vi "总磷单步调试对话框.vi"() -> ()   [LabVIEW 2016, in "斯坦道总磷总氮.lvlib"]
panel:
  in  "单步调试":T9={"注射泵"=enum."注入", "阀口选择"=enum."V1", "灯"=enum."未选择", "ADC值"=enum."未选择", "数值"=4000, "项目输入"=0, "控温"={"氨氮控温"=FALSE, "消解"=FALSE, "恒温"=FALSE, "降温"=FALSE}, "外设选择"={"蠕动泵"=FALSE, "电磁阀1"=FALSE, "电磁阀2"=FALSE, "慢速"=FALSE}, "外设选择2"={"V9-1"=FALSE, "V9-2"=FALSE, "顺时针"=FALSE, "逆时针"=FALSE}, "反滴定"=FALSE, "试剂检测"=FALSE}
  in  "停止":bool
  out "注射器温度":sgl
  out "消解温度":sgl
  out "ADC":sgl
  out "F3":sgl format="%#.6f"
  out "F2":sgl format="%#.6f"
  out "F1":sgl format="%#.6f"
  out "F0":sgl format="%#.6f"
  in  "退出":bool
  in  "启动":bool
  # "单步调试界面"
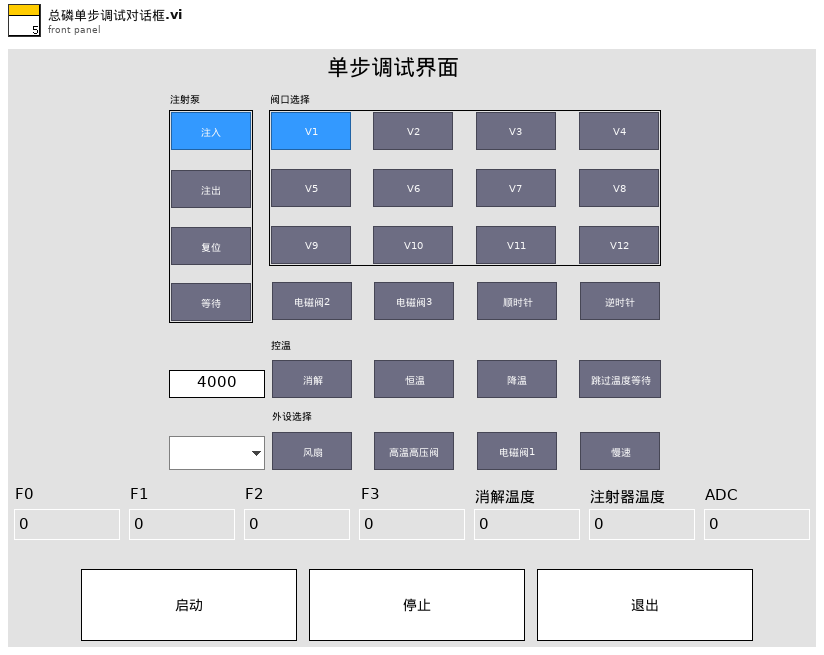
[diagram p1: front panel]
types:
  T1 = typedef "SingleStepTestV3.lvlib/SingleStepTestV3.lvclass/注射泵操作.ctl" = enum32{"复位", "注入", "注出", "等待"}
  T2 = typedef "SingleStepTestV3.lvlib/SingleStepTestV3.lvclass/阀口操作.ctl" = enum32{"未选择", "V1", "V2", "V3", "V4", "V5", "V6", "V7", "V8", "V9", "V10", "V11", "V12"}
  T3 = typedef "SingleStepTestV3.lvlib/SingleStepTestV3.lvclass/灯选择.ctl" = enum32{"未选择", "365", "520", "660", "氙灯/紫灯"}
  T4 = typedef "SingleStepTestV3.lvlib/SingleStepTestV3.lvclass/ADC选择.ctl" = enum32{"未选择", "ADC365", "ADC520", "ADC660", "光谱仪"}
  T5 = typedef "SingleStepTestV3.lvlib/SingleStepTestV3.lvclass/控温操作.ctl" = cluster{"氨氮控温":bool, "消解":bool, "恒温":bool, "降温":bool}
  T6 = typedef "SingleStepTestV3.lvlib/SingleStepTestV3.lvclass/外设选择.ctl" = cluster{"蠕动泵":bool, "电磁阀1":bool, "电磁阀2":bool, "慢速":bool}
  T7 = typedef "SingleStepTestV3.lvlib/SingleStepTestV3.lvclass/外设选择2.ctl" = cluster{"V9-1":bool, "V9-2":bool, "顺时针":bool, "逆时针":bool}
  T8 = typedef "SingleStepTestV3.lvlib/SingleStepTestV3.lvclass/布尔按钮.ctl" = bool
  T9 = cluster{"注射泵":T1, "阀口选择":T2, "灯":T3, "ADC值":T4, "数值":i16, "项目输入":u16, "控温":T5, "外设选择":T6, "外设选择2":T7, "反滴定":T8, "试剂检测":T8}
  T10 = typedef "SingleStepTestV3.lvlib/SingleStepTestV3.lvclass/仪器版本.ctl" = enum16{"V3.1版", "V4版", "V3版", "V4.2版"}
  T11 = typedef "操作日志字段定义.ctl" = cluster{"时间":timestamp, "参数":string, "日志信息":string, "流程参数":string}
  T12 = cluster{"系统时间":timestamp, "工作状态":u16, "测量模式":enum16{"待机", "连续模式", "周期模式", "定点模式", "受控模式", "手动模式"}, "告警代码":u16, "故障代码":u16, "日志代码":u16, "软件版本":u16, "F0":sgl, "F1":sgl, "F2":sgl, "F3":sgl, "T":sgl, "H":sgl, "id":u16, "flowid":u16, "量程":u16, "总磷控温温度1":sgl, "营养盐控温温度2":sgl, "ADC":sgl, "结果值":sgl, "运行时间":u16, "步骤详情":string, "步骤流程":string}
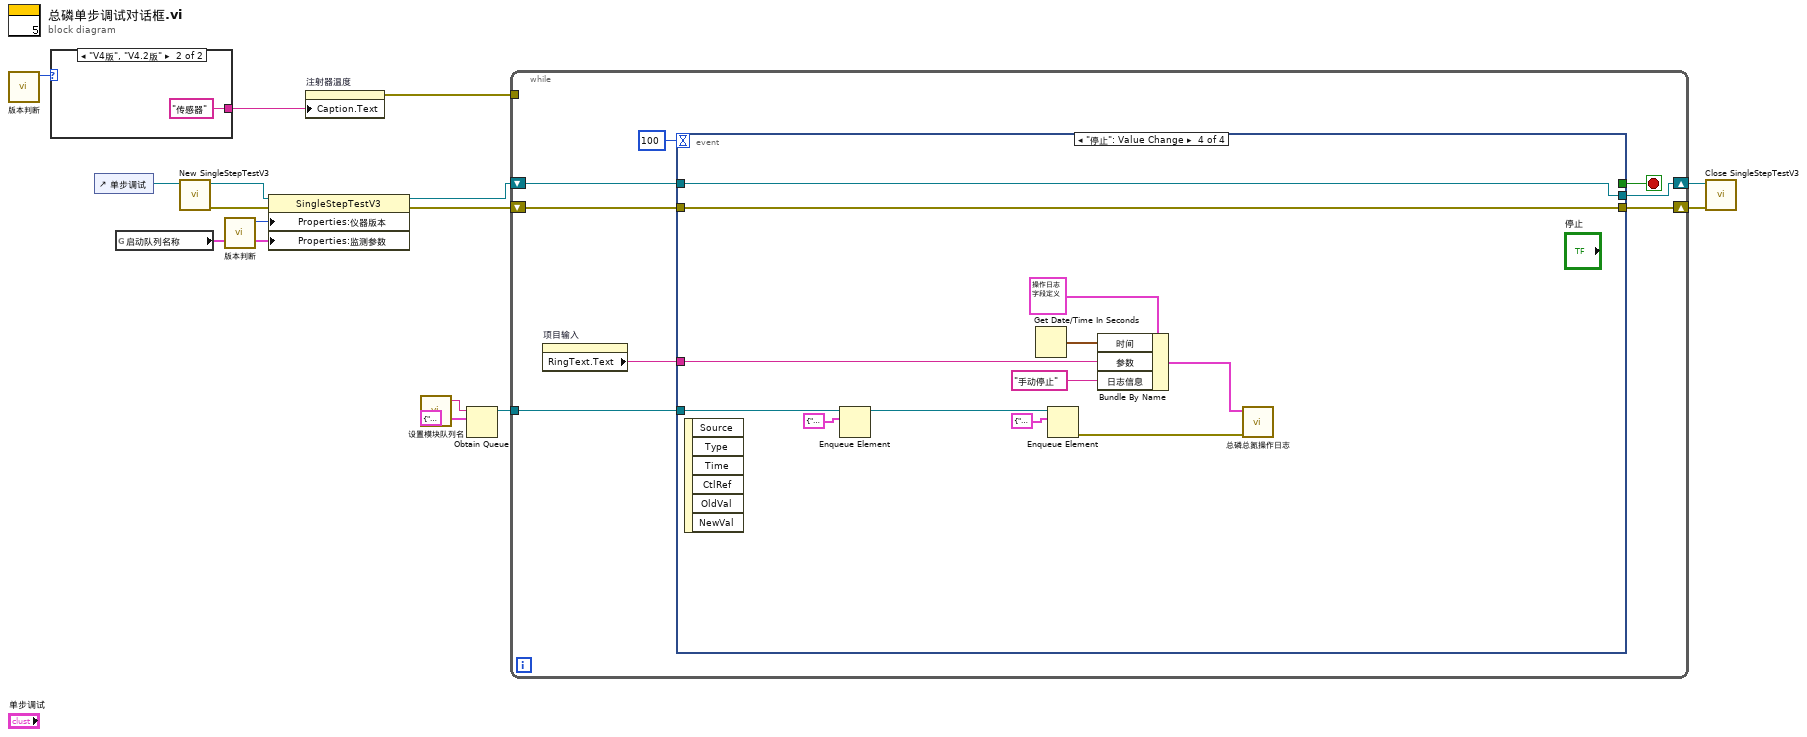
[diagram p0: block diagram]
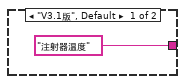
[diagram p2: hidden frame]
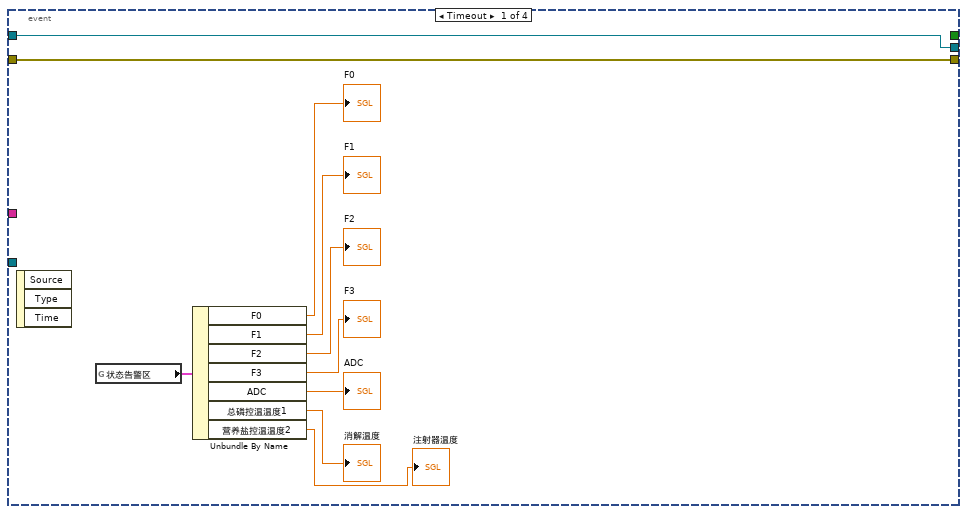
[diagram p3: hidden frame]
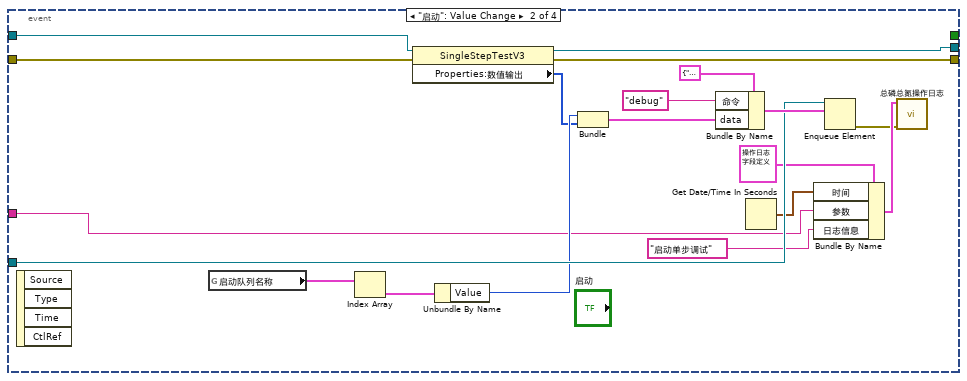
[diagram p4: hidden frame]
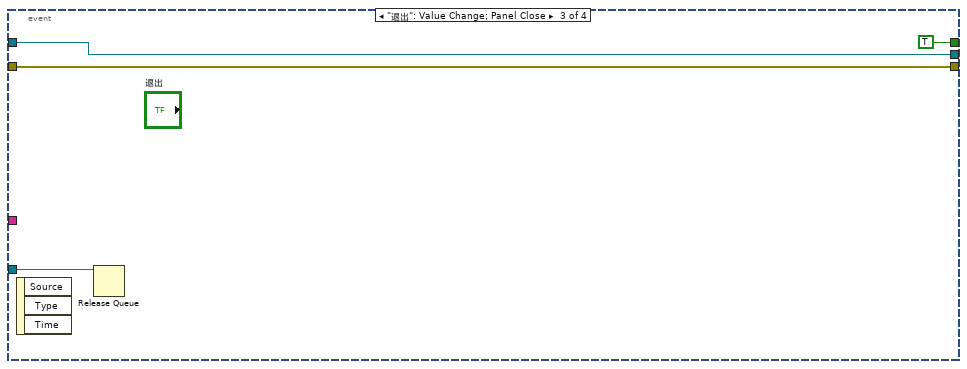
[diagram p5: hidden frame]
diagram:
  n1 = call "版本判断.vi"() -> ("仪器版本"=w12:T10)  [unwired: 11 in]
  n2 = case shown="\"V4版\", \"V4.2版\"" w12 {
    tunnel: ["注射器温度" ("标题.文本") "传感器" ("标题.文本")] -> w11
    frame "V3.1版", Default {
    }
    frame "V4版", "V4.2版" {
    }
  }
  n3 = control-ref of="单步调试"() -> (w1:refnum<vi>)
  n4 = global read "model config var.vi" "启动队列名称"() -> (w2:cluster{"String":string, "Value":u16}[])
  n5 = call "New SingleStepTestV3.vi"("Reference"=w1) -> ("error out"=w5:errorcluster, "SingleStepTestV3 out"=w4:refnum<class "SingleStepTestV3.lvclass">)  [unwired: 9 in]
  n6 = call "版本判断.vi"() -> ("仪器版本"=w3:T10)  [unwired: 11 in]
  n7 = property class="SingleStepTestV3"(reference=w4, error in=w5, "Properties:仪器版本"=w3, "Properties:监测参数"=w2) -> (reference out=w9:refnum<class "SingleStepTestV3.lvclass">, error out=w8:errorcluster)
  n8 = property on="注射器温度" class="DigNum (strict)"("Caption.Text"=w11) -> (error out=w10:errorcluster)  [unwired: 2 in, 1 out]
  n9 = call "设置模块队列名.vi"() -> ("Msg"=w13:string)  [unwired: 5 in]
  n10 = Obtain Queue(name (unnamed)=w13, element data type=cluster{"命令":string, "data":variant} {"命令"="", "data"=variant}) -> (queue out=w14:refnum<queue>)  [unwired: 3 in, 2 out]
  n11 = while {
    tunnel: w14 -> [w25]
    tunnel: w10 -> [_]
    shift-right: [w19] -> w6
    shift-left: w8 -> [w21]
    shift-right: [w20] -> w7
    shift-left: w9 -> [w22]
    stop <- w24 stop-if-true
    n12 = property on="项目输入" class="Ring (strict)"() -> ("RingText.Text"=w18:string)  [unwired: 2 in, 2 out]
    n13 = event shown="[3] \"停止\": Value Change" {
      selector: _ -> [_ _ _ _]
      dyn-events: _ -> [_ _ _ _]
      timeout: 100 -> [_ _ _ _]
      tunnel: w25 -> [_ w50 w57 w67]
      tunnel: [_ _ TRUE _] -> w24
      tunnel: w22 -> [w27 w46 w56 w66]
      tunnel: w21 -> [w26 w45 w55 w65]
      tunnel: [w27 w42 w56 w66] -> w20
      tunnel: [w26 w44 w55 w65] -> w19
      tunnel: w18 -> [_ w36 _ w59]
      event Timeout {
        n14 = event-data() -> ()  [unwired: 1 in, 3 out]
        n15 = global read "VAR总磷总氮全局变量.vi" "状态告警区"() -> (w28:T12)
        n16 = Unbundle By Name(w28) -> ("F0"=→"F0":sgl, "F1"=→"F1":sgl, "F2"=→"F2":sgl, "F3"=→"F3":sgl, "ADC"=→"ADC":sgl, "总磷控温温度1"=→"消解温度":sgl, "营养盐控温温度2"=→"注射器温度":sgl)
      }
      event "启动": Value Change {
        n17 = event-data() -> ()  [unwired: 1 in, 4 out]
        n18 = global read "model config var.vi" "启动队列名称"() -> (w47:cluster{"String":string, "Value":u16}[])
        n19 = Index Array(array=w47) -> (element=w49:cluster{"String":string, "Value":u16})  [unwired: 1 in]
        n20 = property class="SingleStepTestV3"(reference=w46, error in=w45) -> (reference out=w42:refnum<class "SingleStepTestV3.lvclass">, error out=w44:errorcluster, "Properties:数值输出"=w43:u16[])
        n21 = Unbundle By Name(w49) -> ("Value"=w48:u16)
        n22 = Bundle("Value"=w48, "Properties:数值输出"=w43) -> (w51:cluster{"Value":u16, "Properties:数值输出":u16[]})  [unwired: 1 in]
        n23 = Bundle By Name(cluster=cluster{"命令":string, "data":variant} {"命令"="", "data"=variant} ("元素"), "命令"="debug", "data"=w51) -> (w52:cluster{"命令":string, "data":variant})
        n24 = Get Date/Time In Seconds() -> (seconds since 1Jan1904=w39:timestamp)
        n25 = Bundle By Name(cluster=T11 {"时间"=timestamp(0 s since 1904-01-01), "参数"="", "日志信息"="", "流程参数"=""} ("data in"), "时间"=w39, "参数"=w36, "日志信息"="启动单步调试") -> (w40:T11)
        n26 = Enqueue Element(queue=w50, element=w52) -> (error out=w37:errorcluster)  [unwired: 2 in, 2 out]
        n27 = call "总磷总氮操作日志.vi"("错误输入（无错误）"=w37, "data in"=w40) -> ()  [unwired: 9 in, 1 out]
      }
      event "退出": Value Change; Panel Close {
        n28 = event-data() -> ()  [unwired: 1 in, 3 out]
        n29 = Release Queue(queue=w57) -> ()  [unwired: 2 in, 3 out]
      }
      event "停止": Value Change {
        n30 = event-data() -> ()  [unwired: 1 in, 6 out]
        n31 = Enqueue Element(queue=w67, element=cluster{"命令":string, "data":variant} {"命令"="启动", "data"=variant(cluster{"站号":u16, "控制命令输出":u16[]} {"站号"=1, "控制命令输出"=[2816]})} ("元素")) -> (queue out=w68:refnum<queue>)  [unwired: 2 in, 2 out]
        n32 = Get Date/Time In Seconds() -> (seconds since 1Jan1904=w62:timestamp)
        n33 = Enqueue Element(queue=w68, element=cluster{"命令":string, "data":variant} {"命令"="启动", "data"=variant(cluster{"站号":u16, "控制命令输出":u16[]} {"站号"=2, "控制命令输出"=[2816]})} ("元素")) -> (error out=w60:errorcluster)  [unwired: 2 in, 2 out]
        n34 = Bundle By Name(cluster=T11 {"时间"=timestamp(0 s since 1904-01-01), "参数"="", "日志信息"="", "流程参数"=""} ("data in"), "时间"=w62, "参数"=w59, "日志信息"="手动停止") -> (w63:T11)
        n35 = call "总磷总氮操作日志.vi"("错误输入（无错误）"=w60, "data in"=w63) -> ()  [unwired: 9 in, 1 out]
      }
    }
  }
  n36 = call "Close SingleStepTestV3.vi"("error in (no error)"=w6, "SingleStepTestV3 in"=w7) -> ()  [unwired: 9 in, 1 out]
